vi "maszyna stanowa.vi"(9 "Max czas obsługi":dbl, 10 "Queue in":refnum<queue>, 11 "Kasa":T1) -> (2 "Queue in 2":refnum<queue>, 3 "Kasa 2":T1)   [LabVIEW 2014]
doc: "Aktualizuje kasę i kolejkę."
uses:
  Kasy.ctl
  Client.ctl
  LukiBrary.lvlib
panel:
  out "Czas":timestamp[](array[timestamp])
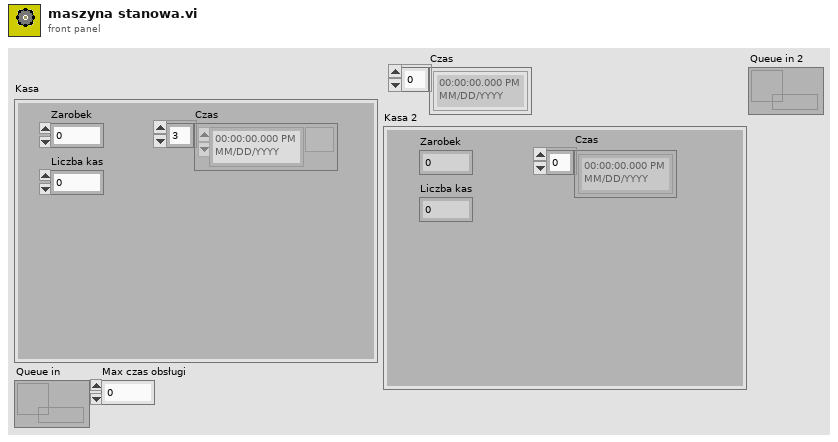
[diagram p1: front panel]
types:
  T1 = typedef "Kasy.ctl" = cluster{"Zarobek":dbl, "Liczba kas":u8, "Czas":timestamp[]}
  T2 = typedef "LukiBrary.lvlib/Client.ctl" = cluster{"Time":dbl, "Price":dbl}
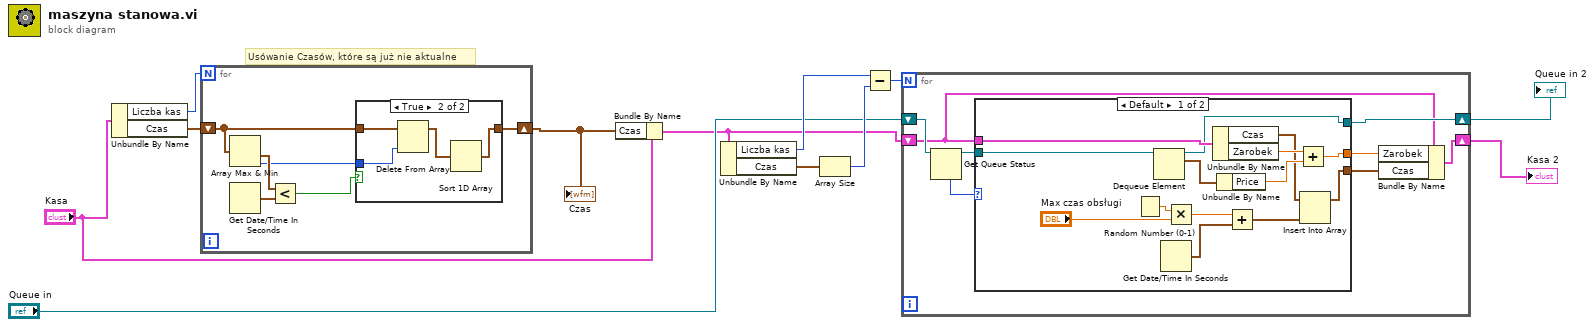
[diagram p0: block diagram]
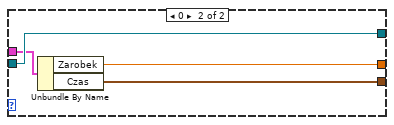
[diagram p2: hidden frame]
diagram:
  # "Usówanie Czasów, które są już nie aktualne"
  n1 = Unbundle By Name("Kasa") -> ("Liczba kas"=w12:u8, "Czas"=w11:timestamp[])
  n2 = for {
    N: w12 -> [_]
    shift-right: [w13] -> w9
    shift-left: w11 -> [w15]
    n3 = Array Max & Min(array=w15) -> (min value=w17:timestamp, min index (indices)=w14:i32)  [unwired: 2 out]
    n4 = Get Date/Time In Seconds() -> (seconds since 1Jan1904=w18:timestamp)
    n5 = Less?(x=w17, y=w18) -> (x < y?=w16:bool)
    n6 = case shown="True" w16 {
      tunnel: w15 -> [w19 w23]
      tunnel: w14 -> [_ w22]
      tunnel: [w19 w20] -> w13
      frame False {
      }
      frame True {
        n7 = Delete From Array(array=w23, index=w22) -> (array with subset deleted=w21:timestamp[])  [unwired: 1 in, 1 out]
        n8 = Sort 1D Array(array=w21) -> (sorted array=w20:timestamp[])
      }
    }
  }
  "Czas" <- w9
  n9 = Bundle By Name(cluster="Kasa", "Czas"=w9) -> (w3:T1)
  n10 = Unbundle By Name(w3) -> ("Liczba kas"=w7:u8, "Czas"=w8:timestamp[])
  n11 = Array Size(array=w8) -> (size(s)=w6:i32)
  n12 = Subtract(x=w7, y=w6) -> (x-y=w5:i32)
  n13 = for {
    N: w5 -> [_]
    shift-right: [w29] -> w1
    shift-left: "Queue in" -> [w31]
    shift-right: [w24] -> w2
    shift-left: w3 -> [w27]
    n14 = Get Queue Status(queue=w31) -> (queue out=w28:refnum<queue>, # elements in queue=w30:i32)  [unwired: 2 in, 6 out]
    n15 = case shown="Default" w30 {
      tunnel: [w43 w49] -> w29
      tunnel: w28 -> [w44 w49]
      tunnel: w27 -> [w45 w48]
      tunnel: [w40 w47] -> w26
      tunnel: [w32 w46] -> w25
      frame Default {
        n16 = Random Number (0-1)() -> (number: 0 to 1=w38:dbl)
        n17 = Dequeue Element(queue=w44) -> (queue out=w43:refnum<queue>, element=w42:T2)  [unwired: 2 in, 2 out]
        n18 = Get Date/Time In Seconds() -> (seconds since 1Jan1904=w35:timestamp)
        n19 = Multiply(x=w38, y="Max czas obsługi") -> (x*y=w36:dbl)
        n20 = Unbundle By Name(w45) -> ("Czas"=w34:timestamp[], "Zarobek"=w41:dbl)
        n21 = Unbundle By Name(w42) -> ("Price"=w39:dbl)
        n22 = Add(x=w36, y=w35) -> (x+y=w33:timestamp)
        n23 = Add(x=w41, y=w39) -> (x+y=w40:dbl)
        n24 = Insert Into Array(array=w34, new element=w33) -> (w32:timestamp[])  [unwired: 1 in]
      }
      frame 0 {
        n25 = Unbundle By Name(w48) -> ("Zarobek"=w47:dbl, "Czas"=w46:timestamp[])
      }
    }
    n26 = Bundle By Name(cluster=w27, "Zarobek"=w26, "Czas"=w25) -> (w24:T1)
  }
  "Kasa 2" <- w2
  "Queue in 2" <- w1
